vi "Simulate Fixed-Point LMS Adaptive Filter.vi"() -> ()   [LabVIEW 2019]
doc: "This example demonstrates how to simulate the performance of a fixed-point LMS adaptive filter. You can try different <b>Step Size</b> values to see how the step size affects the fixed-point conversion. You also can double-click the AFT Simulated Fixed-Point FIR LMS Express VI, located on the block diagram, and experiment with changing the fixed-point settings."
uses:
  <vilib>/addons/Adaptive Filters/Utilities/AFT Fixed-Point Settings.ctl
  <vilib>/addons/Adaptive Filters/Utilities/AFT Algorithm.ctl
  <vilib>/addons/Adaptive Filters/Fixed-Point Simulation/LMS/AFT Simulate Fixed-Point FIR LMS.xnode
  <vilib>/addons/Adaptive Filters/Utilities/AFT Simulation Info.ctl
  <vilib>/addons/Adaptive Filters/NI_AdaptiveFilter.lvlib
panel:
  out "error out":errorcluster
  in  "Save Fixed-Point \nSettings to File":bool
  in  "Step Size":fxp<+/-,16,-2>=0.0019989013671875 format="%#_2f"
  out "Coefficients":dbl[][](graph)
  out "Error Signal":dbl[](graph)
  # "Select Help>>Show Context Help and move the cursor over the VI icon of this example for more information."
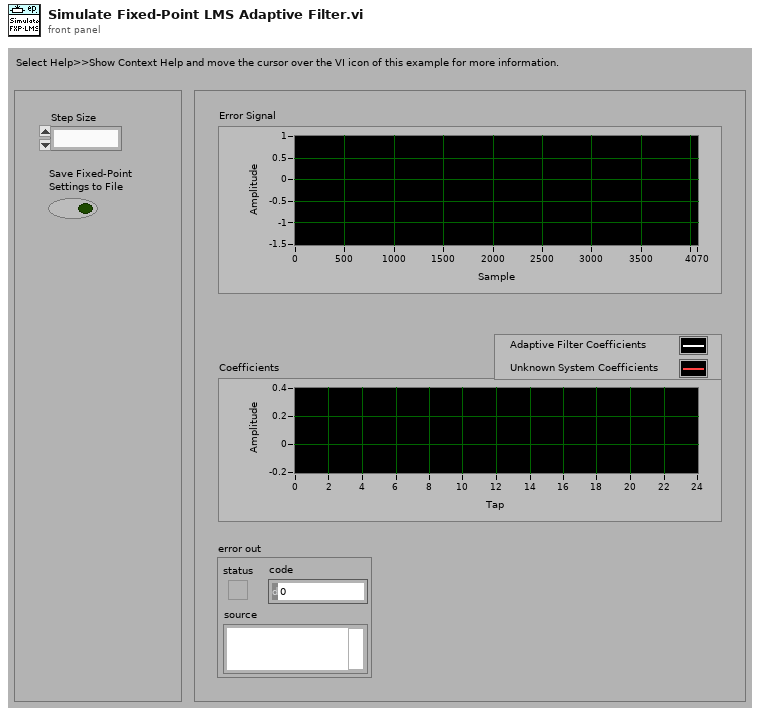
[diagram p1: front panel]
types:
  T1 = typedef "NI_AdaptiveFilter.lvlib/AFT Fixed-Point Settings.ctl" = cluster{"algorithm":u16, "filter length":i32, "step size":dbl, "encoding":cluster{"x(n) word length":i32, "x(n) integer word length":i32, "d(n) word length":i32, "d(n) integer word length":i32, "w(n) word length":i32, "w(n) integer word length":i32, "step size word length":i32, "step size integer word length":i32}}
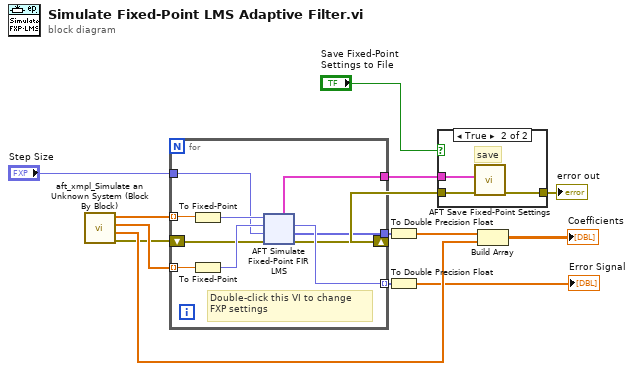
[diagram p0: block diagram]
diagram:
  n1 = call "aft_xmpl_Simulate an Unknown System (Block By Block).vi"() -> ("error out"=w3:errorcluster, "unknown system coefficients"=w14:dbl[], "response signal"=w4:dbl[], "stimulus signal"=w5:dbl[])  [unwired: 4 in, 4 out]
  n2 = for {
    tunnel: w5 -> [w23] mode=indexing
    tunnel: w4 -> [w24] mode=indexing
    tunnel: "Step Size" -> [w20]
    tunnel: [w19] -> w9 mode=indexing
    tunnel: [w18] -> w11
    tunnel: [w17] -> w7
    shift-right: [w16] -> w2
    shift-left: w3 -> [w15]
    # "Double-click this VI to change \nFXP settings"
    n3 = To Fixed-Point(number=w23) -> (fixed-point=w22:fxp<+/-,24,4>)  [unwired: 1 out]
    n4 = To Fixed-Point(number=w24) -> (fixed-point=w21:fxp<+/-,24,4>)  [unwired: 1 out]
    n5 = xnode "AFT Simulate Fixed-Point FIR LMS"("x(n)"=w22, "d(n)"=w21, "step size"=w20, "error in (no error)"=w15) -> ("e(n)"=w19:fxp<+/-,24,4>, "coefficients"=w18:fxp<+/-,24,4>[], "fixed-point settings"=w17:T1, "error out"=w16:errorcluster)  [unwired: 1 in, 2 out]
  }
  n6 = To Double Precision Float(number=w11) -> (double precision float=w10:dbl[])
  n7 = To Double Precision Float(number=w9) -> (double precision float=→"Error Signal":dbl[])
  n8 = case shown="True" "Save Fixed-Point \nSettings to File" {
    tunnel: w7 -> [_ w137]
    tunnel: [w134 w136] -> w1
    tunnel: w2 -> [w134 w135]
    frame False {
    }
    frame True {
      # "save"
      n9 = call <vilib>:"AFT Save Fixed-Point Settings.vi"("error in (no error)"=w135, "fixed-point settings"=w137) -> ("error out"=w136:errorcluster)  [unwired: 1 in, 8 out]
    }
  }
  "error out" <- w1
  n10 = Build Array(w10, w14) -> (→"Coefficients":dbl[][])
